vi "Main.vi"() -> ()   [LabVIEW 2023, in "Application.lvlib"]
doc: "This VI is the main application VI in the Delacor QMH project template. This application VI is implemented as a simple state machine, which communicates with two different Delacor QMH modules.\n_____\nBased on DQMH Project Template 6.1.0.94."
uses:
  Application.lvlib
  Application Data--cluster.ctl
  State--enum.ctl
  <vilib>/Utility/error.llb/DialogType.ctl
  My Cloneable Module/My Cloneable Module.lvlib
  My Singleton Module/My Singleton Module.lvlib
  Chart/Chart.lvlib
  Settings/Settings.lvlib
  DAQ/DAQ.lvlib
  GUI/GUI.lvlib
panel:
  in  "About DQMH":bool
  out "version":string
  in  "Hide My Singleton Module":bool
  in  "Show My Singleton Module":bool
  in  "Hide My Cloneable Module":bool
  in  "Show My Cloneable Module":bool
  in  "Stop My Cloneable Module":bool
  in  "Stop My Singleton Module":bool
  in  "Start My Singleton Module":bool
  out "Active Cloneable Modules":string[](array[string])
  in  "Start New Instance My Cloneable Module":bool
  in  "Select Cloneable Module Instance":i32(ring)=-1 items=["All"=-1]
  in  "My Singleton Module: Do Something Else":dbl caption="Do Something Else"
  in  "My Singleton Module: Do Something":bool
  out "My Singleton Running?":bool
  out "Status":string
  in  "My Cloneable Module: Do Something Else":dbl caption="Do Something Else to Selected Module"
  in  "My Cloneable Module: Do Something":bool caption="Do Something to Selected Module"
  # "This top-level application allows you to launch and control a singleton module, and multiple instances of a cloneable module."
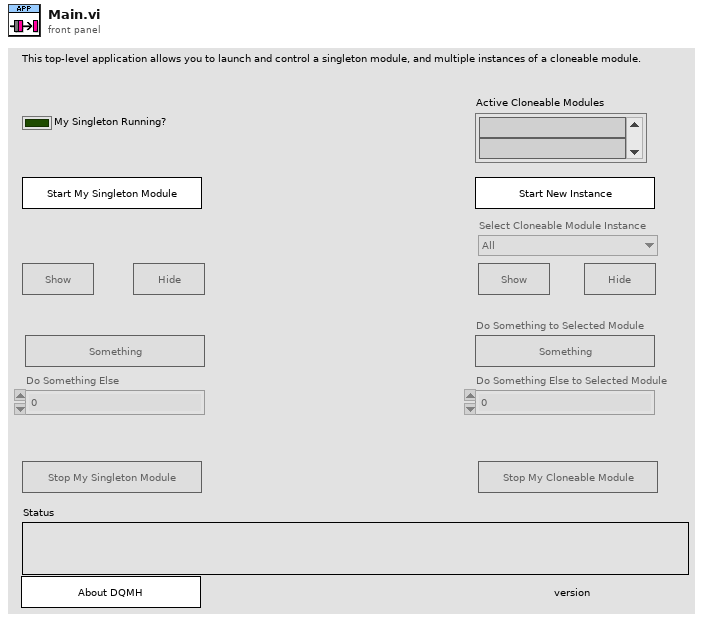
[diagram p1: front panel]
types:
  T1 = typedef "Application.lvlib/State--enum.ctl" = enum16{"Initialize", "Initialize Panel", "Init sub panels", "UI Interlocks", "Update Status", "Wait for Event", "Exit"}
  T2 = typedef "Application.lvlib/Application Data--cluster.ctl" = cluster{"Status":string, "Singleton Controls":refnum<vi>[], "Cloneable Controls":refnum<vi>[], "Module Ring Value":i32}
  T3 = typedef "My Cloneable Module.lvlib/Broadcast Events--cluster.ctl" = cluster{"Module Did Init":refnum<user-event>, "Status Updated":refnum<user-event>, "Error Reported":refnum<user-event>, "Did Something":refnum<user-event>, "Module Did Stop":refnum<user-event>, "Update Module Execution Status":refnum<user-event>}
  T4 = typedef "My Singleton Module.lvlib/Broadcast Events--cluster.ctl" = cluster{"Module Did Init":refnum<user-event>, "Status Updated":refnum<user-event>, "Error Reported":refnum<user-event>, "Did Something":refnum<user-event>, "Module Did Stop":refnum<user-event>, "Update Module Execution Status":refnum<user-event>}
  T5 = enum8{"Enabled", "Disabled", "Disabled and Grayed Out"}
  T6 = typedef "DialogType.ctl" = u16
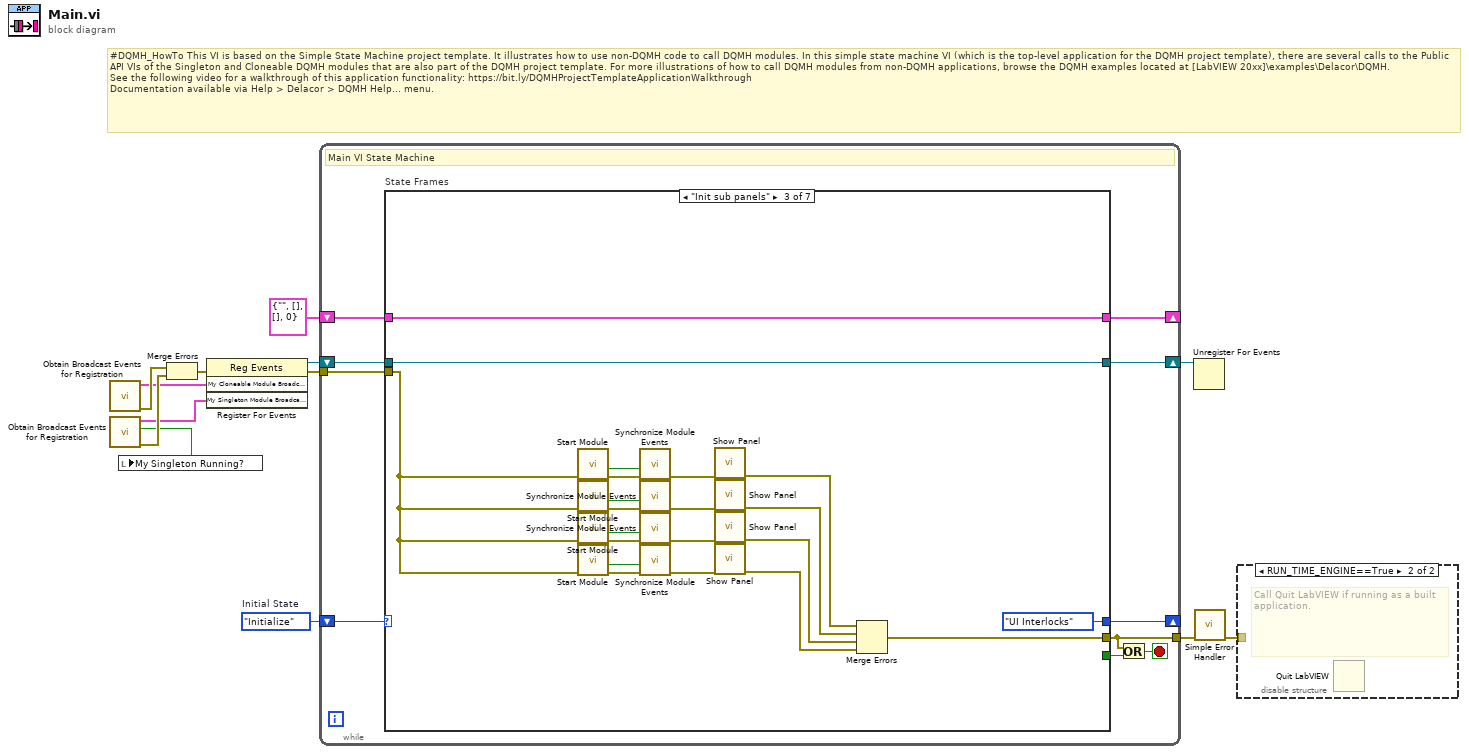
[diagram p0: block diagram]
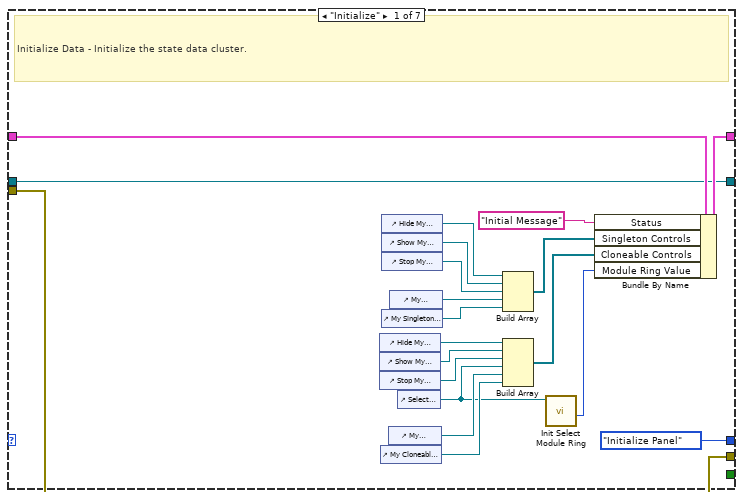
[diagram p2: hidden frame]
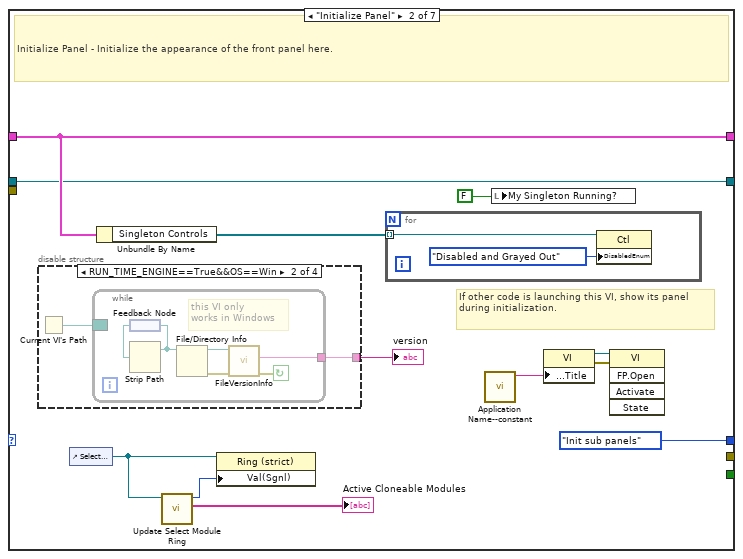
[diagram p3: hidden frame]
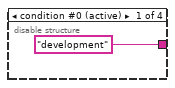
[diagram p4: hidden frame]
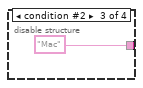
[diagram p5: hidden frame]
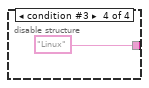
[diagram p6: hidden frame]
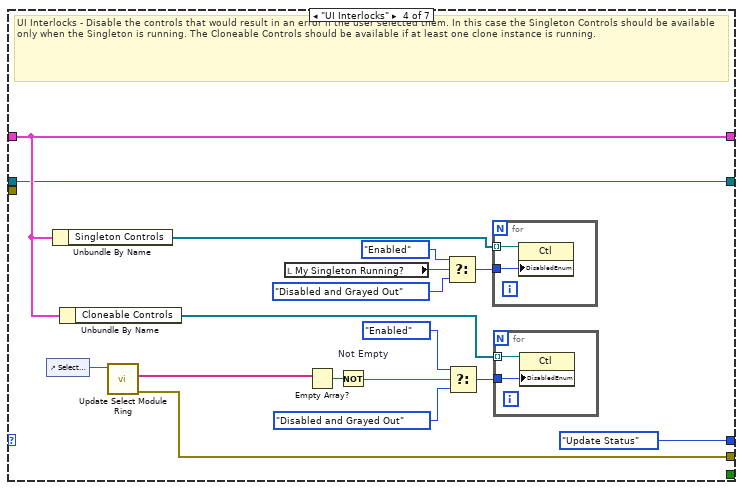
[diagram p7: hidden frame]
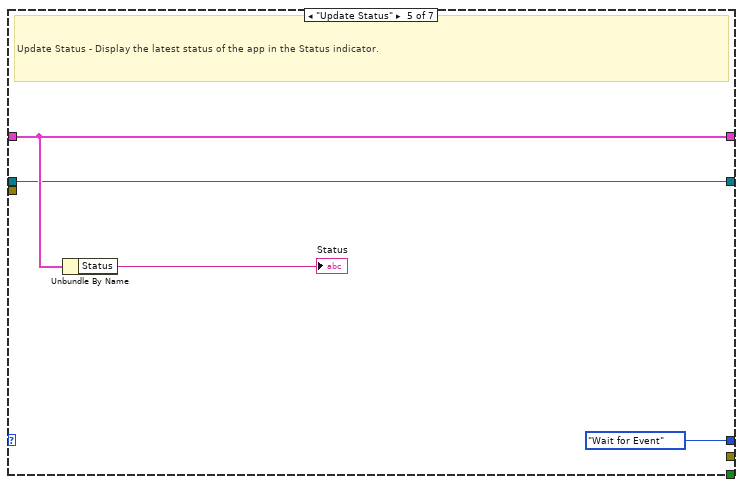
[diagram p8: hidden frame]
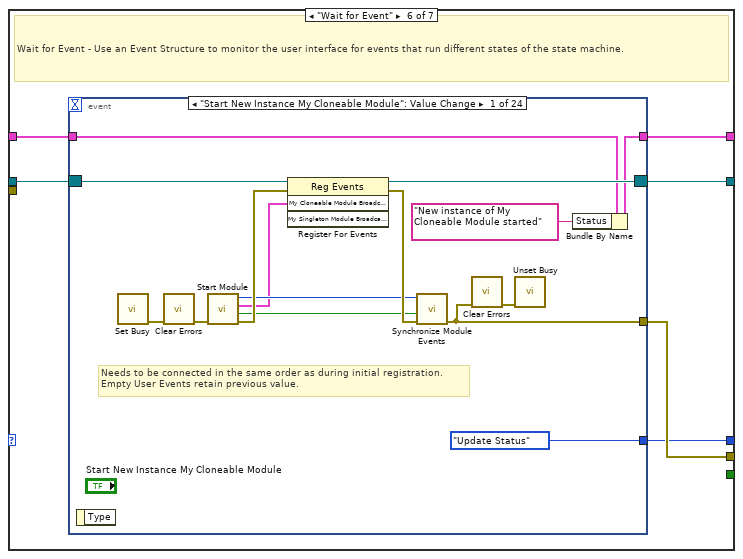
[diagram p9: hidden frame]
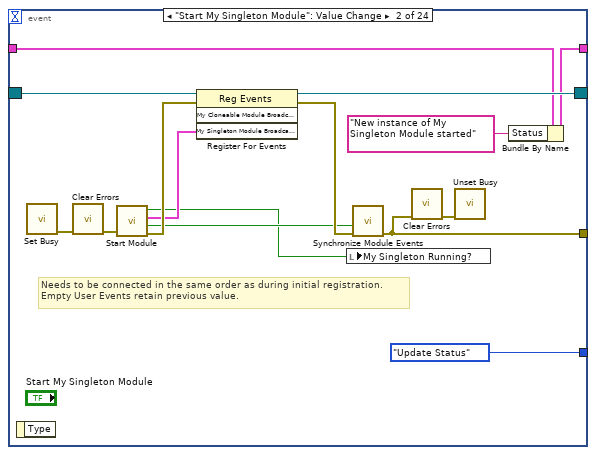
[diagram p10: hidden frame]
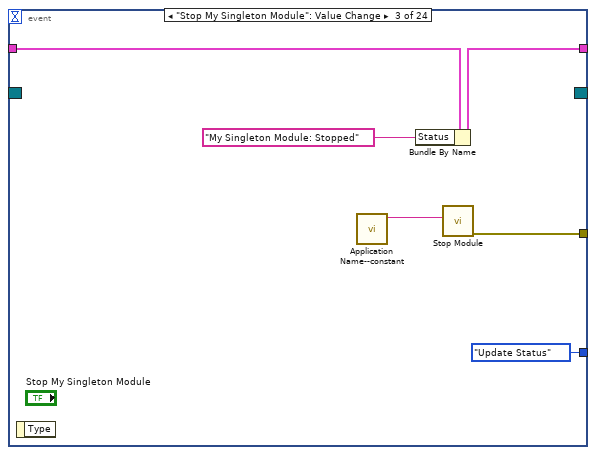
[diagram p11: hidden frame]
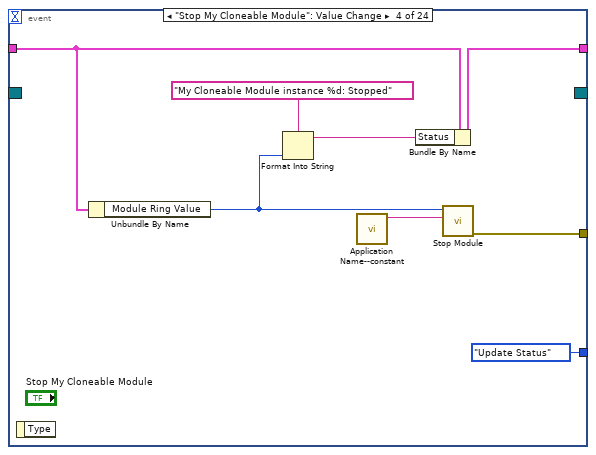
[diagram p12: hidden frame]
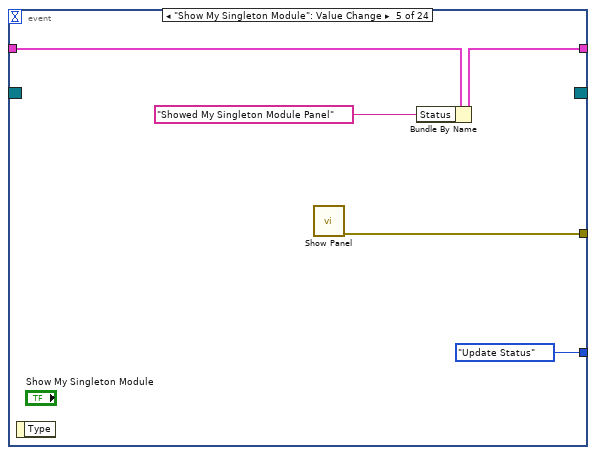
[diagram p13: hidden frame]
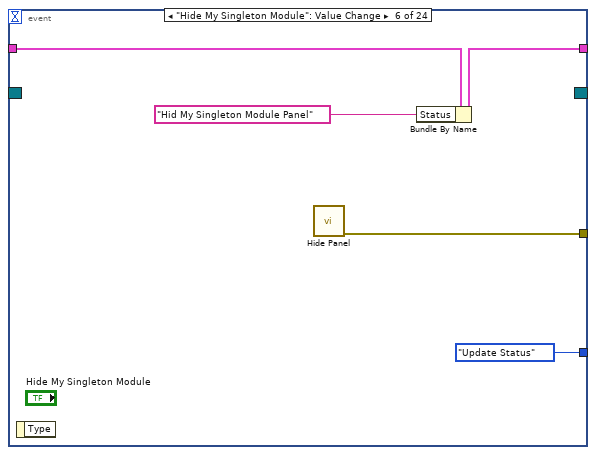
[diagram p14: hidden frame]
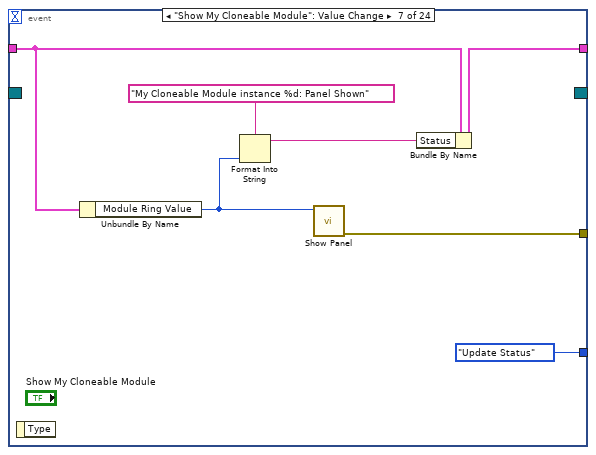
[diagram p15: hidden frame]
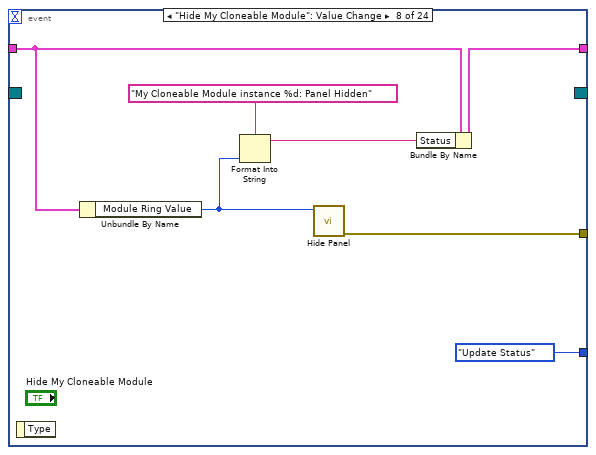
[diagram p16: hidden frame]
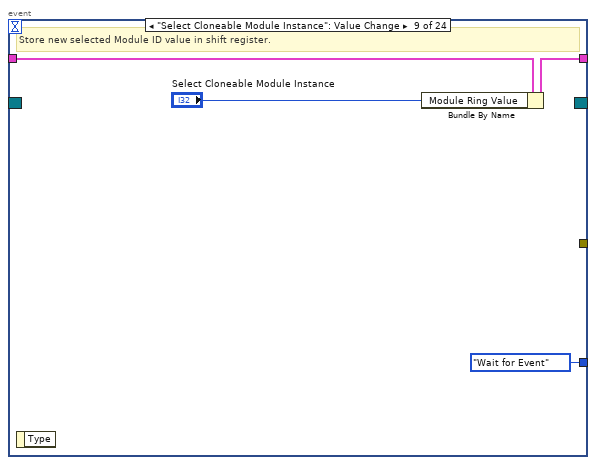
[diagram p17: hidden frame]
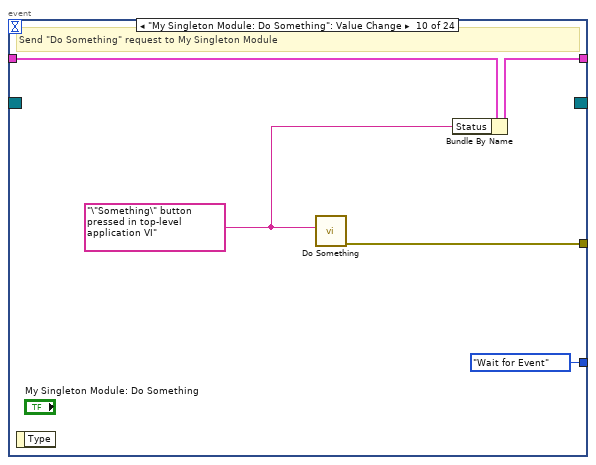
[diagram p18: hidden frame]
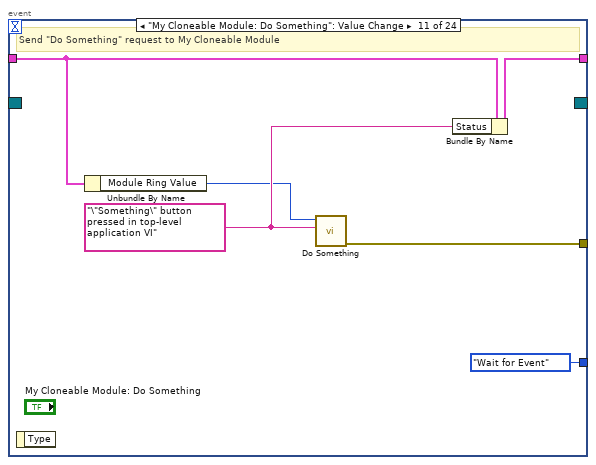
[diagram p19: hidden frame]
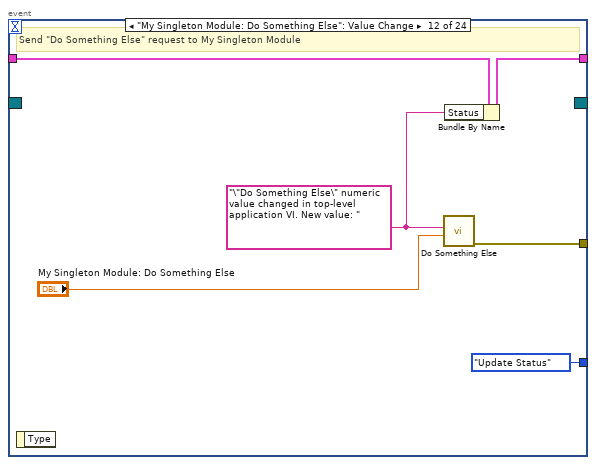
[diagram p20: hidden frame]
diagram:
  w4 = State--enum."Initialize"  # Initial State
  # "#DQMH_HowTo This VI is based on the Simple State Machine project template. It illustrates how to use non-DQMH code to call DQMH modules. In this simple state machine VI (which is the top-level application for the DQMH project template), there are several calls to the Public API VIs of the Singleton and Cloneable DQMH modules that are also part of the DQMH project template. For more illustrations of how to call DQMH modules from non-DQMH applications, browse the DQMH examples located at [LabVIEW 20xx]\\examples\\Delacor\\DQMH.\nSee the following video for a walkthrough of this application functionality: https://bit.ly/DQMHProjectTemplateApplicationWalkthrough\nDocumentation available via Help > Delacor > DQMH Help... menu."
  n1 = call "Obtain Broadcast Events for Registration.vi"() -> ("error out"=w9:errorcluster, "My Cloneable Module Broadcast Events"=w6:T3)  [unwired: 9 in, 1 out]
  n2 = call "Obtain Broadcast Events for Registration.vi"() -> ("error out"=w8:errorcluster, "Already running?"=w1:bool, "My Singleton Module Broadcast Events"=w5:T4)  [unwired: 9 in]
  n3 = local write "My Singleton Running?"(w1) -> ()
  n4 = Merge Errors(w9, w8) -> (w10:errorcluster)
  n5 = register-events(error in=w10, w6, w5) -> (reference out=w3:refnum<event-registration>, error out=w11:errorcluster)  [unwired: 1 in]
  n6 = while {
    shift-right: [w20] -> _
    shift-left: T2 {"Status"="", "Singleton Controls"=[], "Cloneable Controls"=[], "Module Ring Value"=0} ("Data Cluster") -> [w21]
    tunnel: [w23] -> w13
    shift-right: [w16] -> _
    shift-left: w4 -> [w18]
    shift-right: [w14] -> w2
    shift-left: w3 -> [w15]
    tunnel: w11 -> [w22]
    stop <- w17 stop-if-true
    # "Main VI State Machine"
    n7 = case "State Frames" shown="\"Init sub panels\"" w18 {
      tunnel: [w43 _ w77 w106 _ w120 w302] -> w23
      tunnel: w21 -> [w42 w52 w89 w94 w114 w117 w299]
      tunnel: [w41 w52 w89 w94 w114 w116 w299] -> w20
      tunnel: [_ _ _ _ _ _ w298] -> w19
      tunnel: [State--enum."Initialize Panel" ("State") State--enum."Init sub panels" ("State") State--enum."UI Interlocks" ("State") State--enum."Update Status" ("State") State--enum."Wait for Event" ("State") w115 State--enum."Exit" ("State")] -> w16
      tunnel: w15 -> [w24 w49 w88 w90 w111 w119 w296]
      tunnel: [w24 w49 w88 w90 w111 w118 w296] -> w14
      tunnel: w22 -> [w43 _ w86 _ _ _ _]
      frame "Initialize" {
        # "Initialize Data - Initialize the state data cluster."
        n8 = control-ref of="Hide My Cloneable Module"() -> (w33:refnum<vi>)
        n9 = control-ref of="Show My Cloneable Module"() -> (w32:refnum<vi>)
        n10 = control-ref of="Stop My Cloneable Module"() -> (w31:refnum<vi>)
        n11 = control-ref of="My Cloneable Module: Do Something"() -> (w28:refnum<vi>)
        n12 = control-ref of="Hide My Singleton Module"() -> (w39:refnum<vi>)
        n13 = control-ref of="Show My Singleton Module"() -> (w38:refnum<vi>)
        n14 = control-ref of="Stop My Singleton Module"() -> (w37:refnum<vi>)
        n15 = control-ref of="My Singleton Module: Do Something"() -> (w35:refnum<vi>)
        n16 = control-ref of="My Cloneable Module: Do Something Else"() -> (w29:refnum<vi>)
        n17 = control-ref of="My Singleton Module: Do Something Else"() -> (w36:refnum<vi>)
        n18 = control-ref of="Select Cloneable Module Instance"() -> (w26:refnum<vi>)
        n19 = Build Array(w39, w38, w37, w36, w35) -> (w34:refnum<vi>[])
        n20 = Build Array(w33, w32, w31, w26, w29, w28) -> (w30:refnum<vi>[])
        n21 = call "Init Select Module Ring.vi"("Select Module Ring Ref"=w26) -> ("Module Ring Value"=w25:i32)  [unwired: 8 in, 2 out]
        n22 = Bundle By Name(cluster=w42, "Status"="Initial Message" ("Initial Message"), "Singleton Controls"=w34, "Cloneable Controls"=w30, "Module Ring Value"=w25) -> (w41:T2)
      }
      frame "Initialize Panel" {
        # "If other code is launching this VI, show its panel during initialization."
        # "Initialize Panel - Initialize the appearance of the front panel here."
        n23 = disable-structure "Conditional Disable Structure" shown="RUN_TIME_ENGINE==True&&OS==Win" {
          disable-tunnel: ["development" w57 "Mac" "Linux"] -> w46
          frame condition #0 (active) {
          }
          frame condition #1 {
            n24 = Current VI's Path() -> (path=w58:path)
            n25 = while {
              border: w58 -> [_]
              tunnel: [w59] -> w57
              stop <- w63 continue-if-true
              # "this VI only \nworks in Windows"
              n26 = feedback #1() -> (w62:path)
              n27 = Strip Path(path=w62) -> (stripped path=w61:path)  [unwired: 1 out]
              n28 = feedback-in #1(w61) -> ()
              n29 = File/Directory Info(path=w61) -> (path out=w60:path, error out=w64:errorcluster)  [unwired: 1 in, 5 out]
              n30 = call <vilib>:"FileVersionInfo.vi"("error in (no error)"=w64, "Application Path in"=w60) -> ("error out"=w63:errorcluster, "File Version Info"=w59:string)  [unwired: 6 in, 2 out]
            }
          }
          frame condition #2 {
          }
          frame condition #3 {
          }
        }
        "version" <- w46
        n31 = control-ref of="Select Cloneable Module Instance"() -> (w48:refnum<vi>)
        n32 = Unbundle By Name(w52) -> ("Singleton Controls"=w51:refnum<vi>[])
        n33 = call "Update Select Module Ring.vi"("Select Module Ring Ref"=w48) -> ("Active Modules (Array)"=→"Active Cloneable Modules":string[], "New Module Ring Value"=w47:i32)  [unwired: 8 in, 1 out]
        n34 = property on="Property Node" class="Ring (strict)"(reference=w48, "Val(Sgnl)"=w47) -> ()  [unwired: 1 in, 2 out]
        n35 = for {
          tunnel: w51 -> [w68] mode=indexing
          n36 = property on="Property Node" class="Ctl"(reference=w68, "DisabledEnum"=T5."Disabled and Grayed Out" ("Disabled")) -> ()  [unwired: 1 in, 2 out]
        }
        n37 = call "Application Name--constant.vi"() -> ("Application Name"=w45:string)  [unwired: 11 in]
        n38 = local write "My Singleton Running?"(FALSE ("My Singleton Module Init?")) -> ()
        n39 = property on="Property Node" class="VI"("Front Panel.Title"=w45) -> (reference out=w44:refnum<vi>, error out=w55:errorcluster)  [unwired: 2 in]
        n40 = invoke class="VI" method="FP.Open"(reference=w44, error in=w55) -> ()  [unwired: 3 in, 5 out]
      }
      frame "Init sub panels" {
        n41 = call "Start Module.vi"("error in"=w86) -> ("error out"=w79:errorcluster, "Wait for Event Sync?"=w69:bool)  [unwired: 7 in, 2 out]
        n42 = call "Start Module.vi"("error in"=w86) -> ("error out"=w81:errorcluster, "Wait for Event Sync?"=w70:bool)  [unwired: 7 in, 2 out]
        n43 = call "Start Module.vi"("error in"=w86) -> ("error out"=w83:errorcluster, "Wait for Event Sync?"=w71:bool)  [unwired: 7 in, 2 out]
        n44 = call "Start Module.vi"("error in"=w86) -> ("error out"=w85:errorcluster, "Wait for Event Sync?"=w72:bool)  [unwired: 7 in, 2 out]
        n45 = call "Synchronize Module Events.vi"("error in"=w79, "Wait for Event Sync?"=w69) -> ("error out"=w78:errorcluster)  [unwired: 9 in]
        n46 = call "Synchronize Module Events.vi"("error in"=w81, "Wait for Event Sync?"=w70) -> ("error out"=w80:errorcluster)  [unwired: 9 in]
        n47 = call "Synchronize Module Events.vi"("error in"=w83, "Wait for Event Sync?"=w71) -> ("error out"=w82:errorcluster)  [unwired: 9 in]
        n48 = call "Synchronize Module Events.vi"("error in"=w85, "Wait for Event Sync?"=w72) -> ("error out"=w84:errorcluster)  [unwired: 9 in]
        n49 = call "Show Panel.vi"("error in (no error)"=w78) -> ("error out"=w73:errorcluster)  [unwired: 10 in]
        n50 = call "Show Panel.vi"("error in (no error)"=w80) -> ("error out"=w74:errorcluster)  [unwired: 10 in]
        n51 = call "Show Panel.vi"("error in (no error)"=w82) -> ("error out"=w75:errorcluster)  [unwired: 10 in]
        n52 = call "Show Panel.vi"("error in (no error)"=w84) -> ("error out"=w76:errorcluster)  [unwired: 10 in]
        n53 = Merge Errors(w73, w74, w75, w76) -> (w77:errorcluster)
      }
      frame "UI Interlocks" {
        # "UI Interlocks - Disable the controls that would result in an error if the user selected them. In this case the Singleton Controls should be available only when the Singleton is running. The Cloneable Controls should be available if at least one clone instance is running."
        n54 = control-ref of="Select Cloneable Module Instance"() -> (w105:refnum<vi>)
        n55 = Unbundle By Name(w94) -> ("Singleton Controls"=w99:refnum<vi>[])
        n56 = Unbundle By Name(w94) -> ("Cloneable Controls"=w93:refnum<vi>[])
        n57 = call "Update Select Module Ring.vi"("Select Module Ring Ref"=w105) -> ("error out"=w106:errorcluster, "Active Modules (Array)"=w104:string[])  [unwired: 8 in, 1 out]
        n58 = local read "My Singleton Running?"() -> (w98:bool)
        n59 = Empty Array?(array=w104) -> (empty?=w103:bool)
        n60 = Not "Not Empty"(x=w103) -> (.not. x?=w92:bool)
        n61 = Select(t=T5."Enabled" ("Disabled"), s=w98, f=T5."Disabled and Grayed Out" ("Disabled")) -> (s? t:f=w100:T5)
        n62 = Select(t=T5."Enabled" ("Disabled"), s=w92, f=T5."Disabled and Grayed Out" ("Disabled")) -> (s? t:f=w97:T5)
        n63 = for {
          tunnel: w99 -> [w110] mode=indexing
          tunnel: w100 -> [w109]
          n64 = property on="Property Node" class="Ctl"(reference=w110, "DisabledEnum"=w109) -> ()  [unwired: 1 in, 2 out]
        }
        n65 = for {
          tunnel: w93 -> [w108] mode=indexing
          tunnel: w97 -> [w107]
          n66 = property on="Property Node" class="Ctl"(reference=w108, "DisabledEnum"=w107) -> ()  [unwired: 1 in, 2 out]
        }
      }
      frame "Update Status" {
        # "Update Status - Display the latest status of the app in the Status indicator."
        n67 = Unbundle By Name(w114) -> ("Status"=→"Status":string)
      }
      frame "Wait for Event" {
        # "Wait for Event - Use an Event Structure to monitor the user interface for events that run different states of the state machine."
        n68 = event shown="[0] \"Start New Instance My Cloneable Module\": Value Change" {
          selector: w119 -> [w127 w143 _ _ _ _ _ _ _ _ _ _ _ _ _ _ _ _ _ _ _ _ _ _]
          dyn-events: [w126 w142 _ _ _ _ _ _ _ _ _ _ _ _ _ _ _ _ _ _ _ _ _ _] -> w118
          timeout: _ -> [_ _ _ _ _ _ _ _ _ _ _ _ _ _ _ _ _ _ _ _ _ _ _ _]
          tunnel: [w135 w150 w156 w164 w169 w174 w181 w188 _ w197 w203 w209 w216 w224 w229 w233 _ _ _ _ w275 _ _ w286] -> w120
          tunnel: [w122 w139 w152 w161 w167 w172 w180 w187 w190 w195 w202 w207 w215 w218 w226 w232 w235 w240 w255 w264 w268 w279 w284 w288] -> w116
          tunnel: w117 -> [w123 w140 w153 w160 w168 w173 w178 w185 w191 w196 w199 w208 w213 w218 w226 w232 w236 w241 w256 w265 w271 w280 w284 w288]
          tunnel: [State--enum."Update Status" ("State") State--enum."Update Status" ("State") State--enum."Update Status" ("State") State--enum."Update Status" ("State") State--enum."Update Status" ("State") State--enum."Update Status" ("State") State--enum."Update Status" ("State") State--enum."Update Status" ("State") State--enum."Wait for Event" ("State") State--enum."Wait for Event" ("State") State--enum."Wait for Event" ("State") State--enum."Update Status" ("State") State--enum."Update Status" ("State") State--enum."UI Interlocks" ("State") State--enum."UI Interlocks" ("State") State--enum."UI Interlocks" ("State") State--enum."Update Status" ("State") State--enum."Update Status" ("State") State--enum."Update Status" ("State") State--enum."Update Status" ("State") State--enum."UI Interlocks" ("State") State--enum."UI Interlocks" ("State") State--enum."Exit" ("State") State--enum."Wait for Event" ("State")] -> w115
          event "Start New Instance My Cloneable Module": Value Change {
            # "Needs to be connected in the same order as during initial registration.\nEmpty User Events retain previous value."
            n69 = event-data() -> ()  [unwired: 1 in, 1 out]
            n70 = call <vilib>:"Set Busy.vi"() -> ("error out"=w131:errorcluster)  [unwired: 10 in, 1 out]
            n71 = call <vilib>:"Clear Errors.vi"("error in (no error)"=w131) -> ("error out"=w132:errorcluster)  [unwired: 5 in, 1 out]
            n72 = call "Start Module.vi"("error in"=w132) -> ("error out"=w134:errorcluster, "Wait for Event Sync?"=w129:bool, "My Cloneable Module Broadcast Events"=w125:T3, "Module ID"=w128:i32)  [unwired: 7 in]
            n73 = register-events(reference=w127, error in=w134, w125) -> (reference out=w126:refnum<event-registration>, error out=w133:errorcluster)  [unwired: 1 in]
            n74 = call "Synchronize Module Events.vi"("error in"=w133, "Wait for Event Sync?"=w129, "Module ID in"=w128) -> ("error out"=w135:errorcluster)  [unwired: 7 in, 1 out]
            n75 = call <vilib>:"Clear Errors.vi"("error in (no error)"=w135) -> ("error out"=w130:errorcluster)  [unwired: 5 in, 1 out]
            n76 = call <vilib>:"Unset Busy.vi"("error in (no error)"=w130) -> ()  [unwired: 10 in, 1 out]
            n77 = Bundle By Name(cluster=w123, "Status"="New instance of My Cloneable Module started") -> (w122:T2)
          }
          event "Start My Singleton Module": Value Change {
            # "Needs to be connected in the same order as during initial registration.\nEmpty User Events retain previous value."
            n78 = event-data() -> ()  [unwired: 1 in, 1 out]
            n79 = call <vilib>:"Set Busy.vi"() -> ("error out"=w146:errorcluster)  [unwired: 10 in, 1 out]
            n80 = call <vilib>:"Clear Errors.vi"("error in (no error)"=w146) -> ("error out"=w147:errorcluster)  [unwired: 5 in, 1 out]
            n81 = call "Start Module.vi"("error in"=w147) -> ("error out"=w149:errorcluster, "Wait for Event Sync?"=w144:bool, "My Singleton Module Broadcast Events"=w137:T4, "Module Was Already Running?"=w136:bool)  [unwired: 7 in]
            n82 = register-events(reference=w143, error in=w149, w137) -> (reference out=w142:refnum<event-registration>, error out=w148:errorcluster)  [unwired: 1 in]
            n83 = local write "My Singleton Running?"(w136) -> ()
            n84 = call "Synchronize Module Events.vi"("error in"=w148, "Wait for Event Sync?"=w144) -> ("error out"=w150:errorcluster)  [unwired: 9 in]
            n85 = call <vilib>:"Clear Errors.vi"("error in (no error)"=w150) -> ("error out"=w145:errorcluster)  [unwired: 5 in, 1 out]
            n86 = call <vilib>:"Unset Busy.vi"("error in (no error)"=w145) -> ()  [unwired: 10 in, 1 out]
            n87 = Bundle By Name(cluster=w140, "Status"="New instance of My Singleton Module started") -> (w139:T2)
          }
          event "Stop My Singleton Module": Value Change {
            n88 = event-data() -> ()  [unwired: 1 in, 1 out]
            n89 = call "Application Name--constant.vi"() -> ("Application Name"=w154:string)  [unwired: 11 in]
            n90 = Bundle By Name(cluster=w153, "Status"="My Singleton Module: Stopped" ("Message")) -> (w152:T2)
            n91 = call "Stop Module.vi"("Origin"=w154) -> ("error out"=w156:errorcluster)  [unwired: 10 in]
          }
          event "Stop My Cloneable Module": Value Change {
            n92 = event-data() -> ()  [unwired: 1 in, 1 out]
            n93 = Unbundle By Name(w160) -> ("Module Ring Value"=w157:i32)
            n94 = Format Into String(format string="My Cloneable Module instance %d: Stopped" ("Message"), w157) -> (resulting string=w158:string)  [unwired: 2 in, 1 out]
            n95 = call "Application Name--constant.vi"() -> ("Application Name"=w162:string)  [unwired: 11 in]
            n96 = Bundle By Name(cluster=w160, "Status"=w158) -> (w161:T2)
            n97 = call "Stop Module.vi"("Origin"=w162, "Module ID"=w157) -> ("error out"=w164:errorcluster)  [unwired: 9 in]
          }
          event "Show My Singleton Module": Value Change {
            n98 = event-data() -> ()  [unwired: 1 in, 1 out]
            n99 = call "Show Panel.vi"() -> ("error out"=w169:errorcluster)  [unwired: 11 in]
            n100 = Bundle By Name(cluster=w168, "Status"="Showed My Singleton Module Panel" ("Message")) -> (w167:T2)
          }
          event "Hide My Singleton Module": Value Change {
            n101 = event-data() -> ()  [unwired: 1 in, 1 out]
            n102 = call "Hide Panel.vi"() -> ("error out"=w174:errorcluster)  [unwired: 11 in]
            n103 = Bundle By Name(cluster=w173, "Status"="Hid My Singleton Module Panel" ("Message")) -> (w172:T2)
          }
          event "Show My Cloneable Module": Value Change {
            n104 = event-data() -> ()  [unwired: 1 in, 1 out]
            n105 = Unbundle By Name(w178) -> ("Module Ring Value"=w176:i32)
            n106 = Format Into String(format string="My Cloneable Module instance %d: Panel Shown" ("Message"), w176) -> (resulting string=w175:string)  [unwired: 2 in, 1 out]
            n107 = call "Show Panel.vi"("Module ID"=w176) -> ("error out"=w181:errorcluster)  [unwired: 10 in]
            n108 = Bundle By Name(cluster=w178, "Status"=w175) -> (w180:T2)
          }
          event "Hide My Cloneable Module": Value Change {
            n109 = event-data() -> ()  [unwired: 1 in, 1 out]
            n110 = Unbundle By Name(w185) -> ("Module Ring Value"=w183:i32)
            n111 = Format Into String(format string="My Cloneable Module instance %d: Panel Hidden" ("Message"), w183) -> (resulting string=w182:string)  [unwired: 2 in, 1 out]
            n112 = call "Hide Panel.vi"("Module ID"=w183) -> ("error out"=w188:errorcluster)  [unwired: 10 in]
            n113 = Bundle By Name(cluster=w185, "Status"=w182) -> (w187:T2)
          }
          event "Select Cloneable Module Instance": Value Change {
            # "Store new selected Module ID value in shift register."
            n114 = event-data() -> ()  [unwired: 1 in, 1 out]
            n115 = Bundle By Name(cluster=w191, "Module Ring Value"="Select Cloneable Module Instance") -> (w190:T2)
          }
          event "My Singleton Module: Do Something": Value Change {
            w194 = "\"Something\" button pressed in top-level application VI" ("\"Do Something Else\" button pressed")
            # "Send \"Do Something\" request to My Singleton Module"
            n116 = event-data() -> ()  [unwired: 1 in, 1 out]
            n117 = call "Do Something.vi"("Do Something Message"=w194) -> ("error out"=w197:errorcluster)  [unwired: 10 in]
            n118 = Bundle By Name(cluster=w196, "Status"=w194) -> (w195:T2)
          }
          event "My Cloneable Module: Do Something": Value Change {
            w201 = "\"Something\" button pressed in top-level application VI" ("\"Do Something Else\" button pressed")
            # "Send \"Do Something\" request to My Cloneable Module"
            n119 = event-data() -> ()  [unwired: 1 in, 1 out]
            n120 = Unbundle By Name(w199) -> ("Module Ring Value"=w198:i32)
            n121 = call "Do Something.vi"("Do Something Message"=w201, "Module ID"=w198) -> ("error out"=w203:errorcluster)  [unwired: 9 in]
            n122 = Bundle By Name(cluster=w199, "Status"=w201) -> (w202:T2)
          }
          event "My Singleton Module: Do Something Else": Value Change {
            w204 = "\"Do Something Else\" numeric value changed in top-level application VI. New value: " ("\"Do Something Else\" button pressed")
            # "Send \"Do Something Else\" request to My Singleton Module"
            n123 = event-data() -> ()  [unwired: 1 in, 1 out]
            n124 = call "Do Something Else.vi"("X"="My Singleton Module: Do Something Else", "Do Something Else Message"=w204) -> ("error out"=w209:errorcluster)  [unwired: 9 in]
            n125 = Bundle By Name(cluster=w208, "Status"=w204) -> (w207:T2)
          }
          event "My Cloneable Module: Do Something Else": Value Change {
            w210 = "\"Do Something Else\" numeric value changed in top-level application VI. New value: " ("\"Do Something Else\" button pressed")
            # "Send \"Do Something Else\" request to My Cloneable Module"
            n126 = event-data() -> ()  [unwired: 1 in, 1 out]
            n127 = Unbundle By Name(w213) -> ("Module Ring Value"=w212:i32)
            n128 = call "Do Something Else.vi"("X"="My Cloneable Module: Do Something Else", "Do Something else Message"=w210, "Module ID"=w212) -> ("error out"=w216:errorcluster)  [unwired: 8 in]
            n129 = Bundle By Name(cluster=w213, "Status"=w210) -> (w215:T2)
          }
          event User Event {
            # "A new instance of My Cloneable Module has broadcast that is has been initialized"
            n130 = event-data() -> ("Info"=w222:string, "Module ID"=w217:i32)  [unwired: 1 in]
            n131 = local write "Status"(w222) -> ()
            n132 = control-ref of="Select Cloneable Module Instance"() -> (w221:refnum<vi>)
            n133 = call "Update Select Module Ring.vi"("Select Module Ring Ref"=w221) -> ("error out"=w223:errorcluster, "Active Modules (Array)"=w220:string[])  [unwired: 8 in, 1 out]
            n134 = local write "Active Cloneable Modules"(w220) -> ()
            n135 = call "Show Panel.vi"("error in (no error)"=w223, "Module ID"=w217) -> ("error out"=w224:errorcluster)  [unwired: 9 in]
          }
          event User Event {
            # "My Singleton Module has broadcast that it has been initialized"
            n136 = event-data() -> ("Init?"=→"My Singleton Running?":bool, "Info"=w228:string)  [unwired: 1 in]
            n137 = local write "Status"(w228) -> ()
            n138 = call "Show Panel.vi"() -> ("error out"=w229:errorcluster)  [unwired: 11 in]
          }
          event User Event {
            # "My Singleton Module has broadcast its execution status"
            n139 = event-data() -> ("Running?"=w230:bool)  [unwired: 1 in]
            n140 = local write "My Singleton Running?"(w230) -> ()
            n141 = case shown="True" w230 {
              tunnel: [_ w234] -> w233
              frame False {
              }
              frame True {
                n142 = call "Show Panel.vi"() -> ("error out"=w234:errorcluster)  [unwired: 11 in]
              }
            }
          }
          event User Event {
            # "An instance of My Cloneable Module has broadcast its status"
            n143 = event-data() -> ("Status"=w238:string)  [unwired: 1 in]
            n144 = Bundle By Name(cluster=w236, "Status"=w238) -> (w235:T2)
          }
          event User Event {
            # "My Singleton Module has broadcast its status"
            n145 = event-data() -> ("Status"=w242:string)  [unwired: 1 in]
            n146 = Bundle By Name(cluster=w241, "Status"=w242) -> (w240:T2)
          }
          event User Event {
            w247 = T6 0 items=["no dialog", "OK message", "continue or stop message", "OK message + warnings", "continue/stop + warnings"] ("type of dialog (OK msg:1)")
            # "My Cloneable Module had an error"
            n147 = event-data() -> ("Module Name"=w244:string, "Additional Information"=w245:string, "Error"=w246:errorcluster)  [unwired: 1 in]
            n148 = call <vilib>:"Space Constant.vi"() -> ("String"=w251:string)
            n149 = call <vilib>:"Simple Error Handler.vi"("type of dialog (OK msg:1)"=w247, "error in (no error)"=w246) -> ("message"=w248:string)  [unwired: 3 in, 4 out]
            n150 = call <vilib>:"Search and Replace Pattern.vi"("string"=w248, "regular expression (\"\")"="[\\r\\n]" ("regular expression (\"\")"), "replace string (\"\")"=w251, "replace all? (F)"=TRUE ("replace all CR/LF with spaces")) -> ("result string"=w249:string)  [unwired: 1 in, 1 out]
            n151 = Format Into String(format string="%s: %s Additional Information: %s", w244, w249, w245) -> (resulting string=w243:string)  [unwired: 2 in, 1 out]
            n152 = Bundle By Name(cluster=w256, "Status"=w243) -> (w255:T2)
          }
          event User Event {
            # "My Singleton Module had an error"
            n153 = event-data() -> ("Module Name"=w258:string, "Additional Information"=w262:string, "Error"=w266:errorcluster)  [unwired: 1 in]
            n154 = Unbundle By Name(w266) -> ("code"=w257:i32, "source"=w261:string)
            n155 = Format Into String(format string="Error code %d Module: %s  Additional Information: %s\nSource: %s", w257, w258, w262, w261) -> (resulting string=w259:string)  [unwired: 2 in, 1 out]
            n156 = Bundle By Name(cluster=w265, "Status"=w259) -> (w264:T2)
          }
          event User Event {
            n157 = event-data() -> ("Origin"=w270:string)  [unwired: 1 in]
            n158 = Bundle By Name(cluster=w271, "Status"=w270) -> (w269:T2)
            n159 = control-ref of="Select Cloneable Module Instance"() -> (w274:refnum<vi>)
            n160 = call "Update Select Module Ring.vi"("Select Module Ring Ref"=w274) -> ("error out"=w275:errorcluster, "Active Modules (Array)"=w273:string[], "New Module Ring Value"=w267:i32)  [unwired: 8 in]
            n161 = Bundle By Name(cluster=w269, "Module Ring Value"=w267) -> (w268:T2)
            n162 = local write "Active Cloneable Modules"(w273) -> ()
          }
          event User Event {
            n163 = event-data() -> ("Origin"=w277:string)  [unwired: 1 in]
            n164 = local write "My Singleton Running?"(FALSE ("My Singleton Module Init?")) -> ()
            n165 = Concatenate Strings(w277, " Did Stop.") -> (w276:string)
            n166 = Bundle By Name(cluster=w280, "Status"=w276) -> (w279:T2)
          }
          event Panel Close? {
            # "Go to the 'Exit' state if the user tries to close the panel."
            n167 = event-data() -> ()  [unwired: 1 in, 1 out]
            n168 = event-data ("Event Filter Node")("Discard?"=TRUE) -> ()  [unwired: 1 in, 1 out]
          }
          event "About DQMH": Value Change {
            # "Display DQMH About Box"
            n169 = event-data() -> ()  [unwired: 1 in, 1 out]
            n170 = call <vilib>:"DQMH_About Box.vi"() -> ("error out"=w286:errorcluster)  [unwired: 11 in]
          }
        }
      }
      frame "Exit" {
        w293 = TRUE  # Wait for Module to stop?
        w298 = TRUE  # Stop the VI
        # "Stop all modules launched"
        # "Exit - Exit the application."
        n171 = call "Application Name--constant.vi"() -> ("Application Name"=w294:string)  [unwired: 11 in]
        n172 = call "Stop Module.vi"("Wait for Module to stop? (F)"=w293, "Origin"=w294, "Module ID"=-1) -> ("error out"=w300:errorcluster)  [unwired: 8 in]
        n173 = call "Stop Module.vi"("Wait for Module to Stop? (F)"=w293, "Origin"=w294) -> ("error out"=w301:errorcluster)  [unwired: 9 in]
        n174 = call "Stop Module.vi"() -> ("error out"=w289:errorcluster)  [unwired: 11 in]
        n175 = call "Stop Module.vi"() -> ("error out"=w290:errorcluster)  [unwired: 11 in]
        n176 = call "Stop Module.vi"() -> ("error out"=w291:errorcluster)  [unwired: 11 in]
        n177 = call "Stop Module.vi"() -> ("error out"=w292:errorcluster)  [unwired: 11 in]
        n178 = Merge Errors(w289, w290, w291, w292, w300, w301) -> (w302:errorcluster)
      }
    }
    n179 = Or(x=w23, y=w19) -> (x .or. y?=w17:bool)
  }
  n180 = Unregister For Events(event registration refnum=w2) -> ()  [unwired: 1 in, 1 out]
  n181 = call <vilib>:"Simple Error Handler.vi"("error in (no error)"=w13) -> ("error out"=w12:errorcluster)  [unwired: 4 in, 4 out]
  n182 = disable-structure "Conditional Disable Structure" shown="RUN_TIME_ENGINE==True" {
    disable-tunnel: w12 -> [_ _]
    frame condition #0 (active) {
    }
    frame condition #1 {
      # "Call Quit LabVIEW if running as a built application."
      n183 = Quit LabVIEW() -> ()  [unwired: 1 in]
    }
  }
